vi "GetProduct.vi"(8 "error in":errorcluster, 11 "Creator":refnum<class "Creator.lvclass">) -> (0 "error out":errorcluster, 2 "Product":refnum<class "Product.lvclass">, 3 "Creator":refnum<class "Creator.lvclass">)   [LabVIEW 2020, in "FactoryMethod.lvlib" / "FactoryMethodLazyEvaluation.lvlib" / "Creator.lvclass"]
uses:
  Creator.lvclass
  Product/Product.lvclass
  Creator.lvclass/Creator.ctl
  Private/Property/Product/Write Product.vi
  Private/Property/Product/Read Product.vi
  Support/Class/ConsoleOutput.lvclass
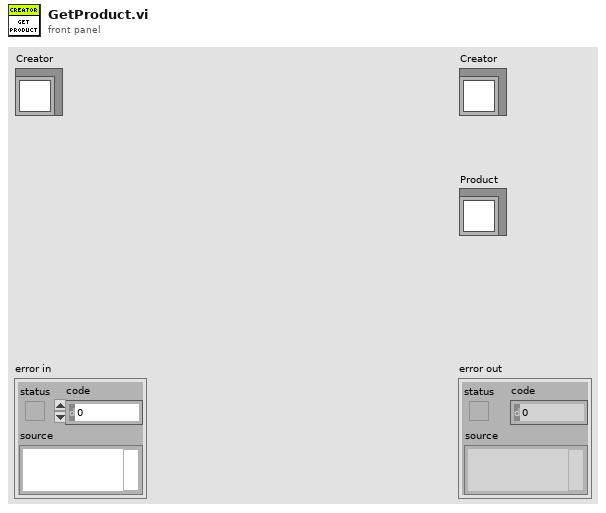
[diagram p1: front panel]
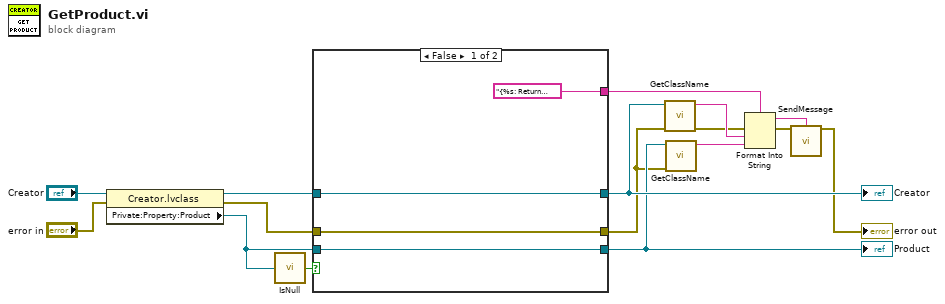
[diagram p0: block diagram]
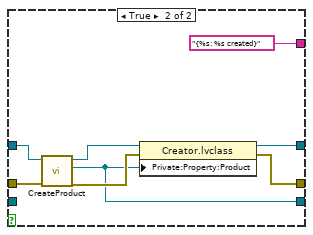
[diagram p2: hidden frame]
diagram:
  n1 = property class="Creator.lvclass"(reference="Creator", error in="error in") -> (reference out=w14:refnum<class "Creator.lvclass">, error out=w12:errorcluster, "Private:Property:Product"=w11:refnum<class "Product.lvclass">)
  n2 = call-dynamic "IsNull.vi"("IDisposable"=w11) -> ("isNull"=w15:bool)  [unwired: 4 in]
  n3 = case shown="False" w15 {
    tunnel: w14 -> [w20 w27]
    tunnel: w12 -> [w18 w26]
    tunnel: [w20 w28] -> w8
    tunnel: [w19 w23] -> w7
    tunnel: w11 -> [w19 _]
    tunnel: [w18 w25] -> w4
    tunnel: ["{%s: Return %s}" ("Message") "{%s: %s created}" ("Message")] -> w1
    frame False {
    }
    frame True {
      n4 = call-dynamic "CreateProduct.vi"("error in (no error)"=w26, "Creator"=w27) -> ("error out"=w24:errorcluster, "Product"=w23:refnum<class "Product.lvclass">, "Creator"=w22:refnum<class "Creator.lvclass">)  [unwired: 7 in]
      n5 = property class="Creator.lvclass"(reference=w22, error in=w24, "Private:Property:Product"=w23) -> (reference out=w28:refnum<class "Creator.lvclass">, error out=w25:errorcluster)
    }
  }
  "Creator" <- w8
  "Product" <- w7
  n6 = call "GetClassName.vi"("error in (no error)"=w4, "object"=w8) -> ("error out"=w3:errorcluster, "Class Name"=w6:string)  [unwired: 8 in]
  n7 = call "GetClassName.vi"("error in (no error)"=w4, "object"=w7) -> ("Class Name"=w5:string)  [unwired: 8 in, 1 out]
  n8 = Format Into String(format string=w1, error in=w3, w6, w5) -> (resulting string=w9:string, error out=w10:errorcluster)  [unwired: 1 in]
  n9 = call "SendMessage.vi"("Message"=w9, "error in (no error)"=w10) -> ("error out"=→"error out":errorcluster)  [unwired: 13 in]
